vi "Html Report.vi"(0 "标题配置":cluster{"title":string, "font":T1}={"title"="测试报告", "font"={"font name"="", "font size"=24.0, "bold"=2, "italic"=2, "underline"=2, "strike through"=2, "font color"=16777222}} {"font"."font size" format="%0.2f"; "font"."strike through" items=["Unchanged", "Yes", "No"]; "font"."underline" items=["Unchanged", "Yes", "No"]; "font"."italic" items=["Unchanged", "Yes", "No"]; "font"."bold" items=["Unchanged", "Yes", "No"]}, 1 "测试信息":cluster{"font":T1, "字符串":string}={"font"={"font name"="", "font size"=12.0, "bold"=2, "italic"=2, "underline"=2, "strike through"=2, "font color"=16777222}, "字符串"=""} {"font"."font size" format="%0.2f"; "font"."strike through" items=["Strk Unchanged", "Strk Yes", "Strk No"]; "font"."underline" items=["Und Unchanged", "Und Yes", "Und No"]; "font"."italic" items=["Ital Unchanged", "Ital Yes", "Ital No"]; "font"."bold" items=["Bold Unchanged", "Bold Yes", "Bold No"]}, 2 "文本":cluster{"font":T1, "字符串":string}={"font"={"font name"="", "font size"=12.0, "bold"=2, "italic"=2, "underline"=2, "strike through"=2, "font color"=16777222}, "字符串"=""} {"font"."font size" format="%0.2f"; "font"."strike through" items=["Strk Unchanged", "Strk Yes", "Strk No"]; "font"."underline" items=["Und Unchanged", "Und Yes", "Und No"]; "font"."italic" items=["Ital Unchanged", "Ital Yes", "Ital No"]; "font"."bold" items=["Bold Unchanged", "Bold Yes", "Bold No"]}, 3 "表格":T2={"auto format"=11, "font"={"font name"="", "font size"=0.0, "bold"=0, "italic"=0, "underline"=0, "strike through"=0, "font color"=0}, "表格 2"=[["1", "1.5", "5.6", "5.6", "7.9", "4.6"], ["2", "2.5", "7.6", "6.5", "7.2", "7.5"], ["3", "6.8", "9.1", "4.2", "6.2", "6.1"], ["4", "6.7", "7.1", "7.2", "1.0", "8.3"], ["5", "6.4", "4.3", "9.2", "5.8", "4.2"], ["6", "8.6", "8.2", "4.3", "8.6", "4.5"]]} {"auto format" items=["xlRangeAutoFormat3DEffects1"=13, "xlRangeAutoFormat3DEffects2"=14, "xlRangeAutoFormatAccounting1"=4, "xlRangeAutoFormatAccounting2"=5, "xlRangeAutoFormatAccounting3"=6, "xlRangeAutoFormatAccounting4"=17, "xlRangeAutoFormatClassic1"=1, "xlRangeAutoFormatClassic2"=2, "xlRangeAutoFormatClassic3"=3, "xlRangeAutoFormatColor1"=7, "xlRangeAutoFormatColor2"=8, "xlRangeAutoFormatColor3"=9, "xlRangeAutoFormatList1"=10, "xlRangeAutoFormatList2"=11, "xlRangeAutoFormatList3"=12, "xlRangeAutoFormatLocalFormat1"=15, "xlRangeAutoFormatLocalFormat2"=16, "xlRangeAutoFormatLocalFormat3"=19, "xlRangeAutoFormatLocalFormat4"=20, "xlRangeAutoFormatReport1"=21, "xlRangeAutoFormatReport2"=22, "xlRangeAutoFormatReport3"=23, "xlRangeAutoFormatReport4"=24, "xlRangeAutoFormatReport5"=25, "xlRangeAutoFormatReport6"=26, "xlRangeAutoFormatReport7"=27, "xlRangeAutoFormatReport8"=28, "xlRangeAutoFormatReport9"=29, "xlRangeAutoFormatReport10"=30, "xlRangeAutoFormatClassicPivotTable"=31, "xlRangeAutoFormatTable1"=32, "xlRangeAutoFormatTable2"=33, "xlRangeAutoFormatTable3"=34, "xlRangeAutoFormatTable4"=35, "xlRangeAutoFormatTable5"=36, "xlRangeAutoFormatTable6"=37, "xlRangeAutoFormatTable7"=38, "xlRangeAutoFormatTable8"=39, "xlRangeAutoFormatTable9"=40, "xlRangeAutoFormatTable10"=41, "xlRangeAutoFormatPTNone"=42, "xlRangeAutoFormatNone"=-4142, "xlRangeAutoFormatSimple"=-4154]; "font"."font size" format="%0.2f"; "font"."strike through" items=["Strk Unchanged", "Strk Yes", "Strk No"]; "font"."underline" items=["Und Unchanged", "Und Yes", "Und No"]; "font"."italic" items=["Ital Unchanged", "Ital Yes", "Ital No"]; "font"."bold" items=["Bold Unchanged", "Bold Yes", "Bold No"]}, 4 "图表配置":T4={"chart type"=4, "graph title (\"\")"="测试图表"} {"chart type" items=["xlColumnClustered"=51, "xlColumnStacked"=52, "xlColumnStacked100"=53, "xl3DColumnClustered"=54, "xl3DColumnStacked"=55, "xl3DColumnStacked100"=56, "xlBarClustered"=57, "xlBarStacked"=58, "xlBarStacked100"=59, "xl3DBarClustered"=60, "xl3DBarStacked"=61, "xl3DBarStacked100"=62, "xlLineStacked"=63, "xlLineStacked100"=64, "xlLineMarkers"=65, "xlLineMarkersStacked"=66, "xlLineMarkersStacked100"=67, "xlPieOfPie"=68, "xlPieExploded"=69, "xl3DPieExploded"=70, "xlBarOfPie"=71, "xlXYScatterSmooth"=72, "xlXYScatterSmoothNoMarkers"=73, "xlXYScatterLines"=74, "xlXYScatterLinesNoMarkers"=75, "xlAreaStacked"=76, "xlAreaStacked100"=77, "xl3DAreaStacked"=78, "xl3DAreaStacked100"=79, "xlDoughnutExploded"=80, "xlRadarMarkers"=81, "xlRadarFilled"=82, "xlSurface"=83, "xlSurfaceWireframe"=84, "xlSurfaceTopView"=85, "xlSurfaceTopViewWireframe"=86, "xlBubble"=15, "xlBubble3DEffect"=87, "xlStockHLC"=88, "xlStockOHLC"=89, "xlStockVHLC"=90, "xlStockVOHLC"=91, "xlCylinderColClustered"=92, "xlCylinderColStacked"=93, "xlCylinderColStacked100"=94, "xlCylinderBarClustered"=95, "xlCylinderBarStacked"=96, "xlCylinderBarStacked100"=97, "xlCylinderCol"=98, "xlConeColClustered"=99, "xlConeColStacked"=100, "xlConeColStacked100"=101, "xlConeBarClustered"=102, "xlConeBarStacked"=103, "xlConeBarStacked100"=104, "xlConeCol"=105, "xlPyramidColClustered"=106, "xlPyramidColStacked"=107, "xlPyramidColStacked100"=108, "xlPyramidBarClustered"=109, "xlPyramidBarStacked"=110, "xlPyramidBarStacked100"=111, "xlPyramidCol"=112, "xl3DColumn"=-4100, "xlLine"=4, "xl3DLine"=-4101, "xl3DPie"=-4102, "xlPie"=5, "xlXYScatter"=-4169, "xl3DArea"=-4098, "xlArea"=1, "xlDoughnut"=-4120, "xlRadar"=-4151]}, 6 "报告类型":u16(ring)=2, 7 "簇":T3={"Save Report 2"=FALSE, "路径"=path "/Report.html", "Print Report 2"=FALSE, "份数"=1} {"份数" min=1 max=10 step=1}) -> ()   [LabVIEW 2014]
uses:
  <vilib>/addons/_office/_wordsub.llb/font.ctl
  <vilib>/Utility/NIReport.llb/Append Report Text (str wrap).vi
  <vilib>/printing/OpenHTMLReport.llb/Open HTML Report in Browser (Refnum).vi
  <vilib>/Utility/NIReport.llb/NI_report.lvclass
  <vilib>/Utility/NIReport.llb/NI_ReportGenerationCore.lvlib
panel:
  out "表格 2":string[][](table)=[["1", "1.5", "5.6", "5.6", "7.9", "4.6"], ["2", "2.5", "7.6", "6.5", "7.2", "7.5"], ["3", "6.8", "9.1", "4.2", "6.2", "6.1"], ["4", "6.7", "7.1", "7.2", "1.0", "8.3"], ["5", "6.4", "4.3", "9.2", "5.8", "4.2"], ["6", "8.6", "8.2", "4.3", "8.6", "4.5"]]
  out "波形图":i32[][](graph)
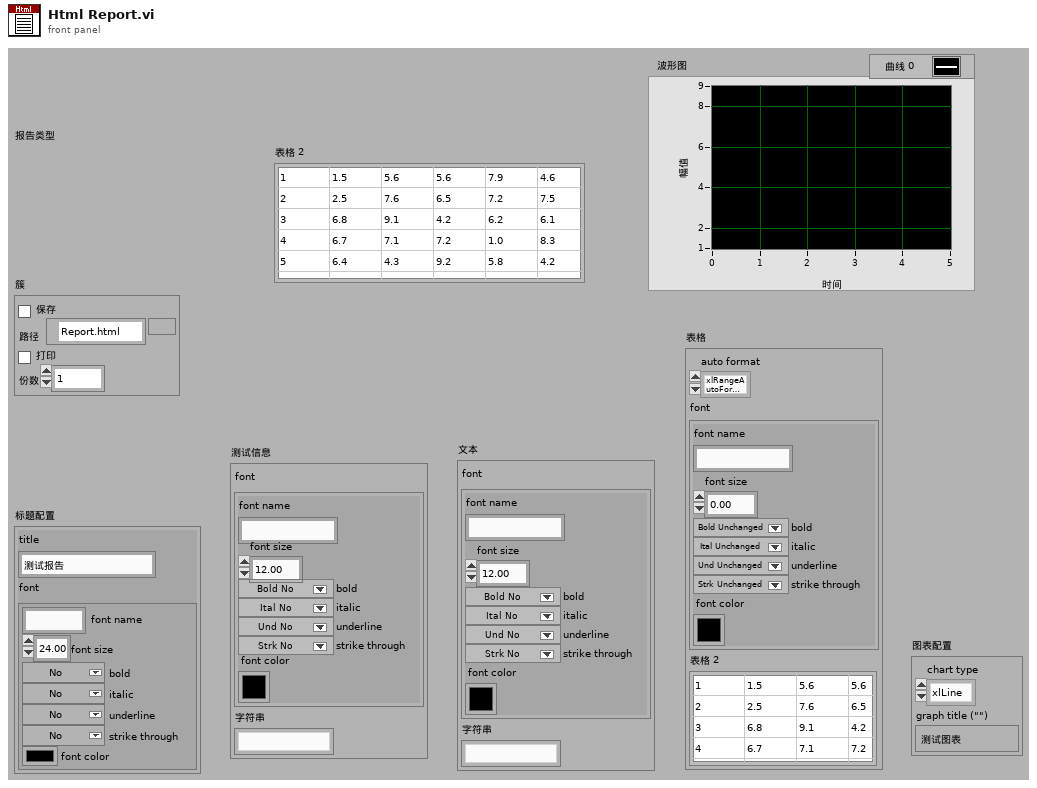
[diagram p1: front panel]
types:
  T1 = typedef "font.ctl" = cluster{"font name":string, "font size":dbl, "bold":u16, "italic":u16, "underline":u16, "strike through":u16, "font color":u32}
  T2 = cluster{"auto format":i32, "font":T1, "表格 2":string[][]}
  T3 = cluster{"Save Report 2":bool, "路径":path, "Print Report 2":bool, "份数":i32}
  T4 = cluster{"chart type":i32, "graph title (\"\")":string}
  T5 = cluster{"Charset (-1)":i16, "Weight (-1)":i16, "Name":string, "Size":string}
  T6 = cluster{"Italic":enum16{"Italic Unchanged", "Italic On", "Italic Off"}, "Strike Through":enum16{"Strike Through Unchanged", "Strike Through On", "Strike Through Off"}, "Underline":enum16{"Underline Unchanged", "Underline On", "Underline Off"}, "Bold":enum16{"Bold Unchanged", "Bold On", "Bold Off"}}
  T7 = typedef "Generate Report Object Reference.ctl" = refnum<class "NI_report.lvclass">
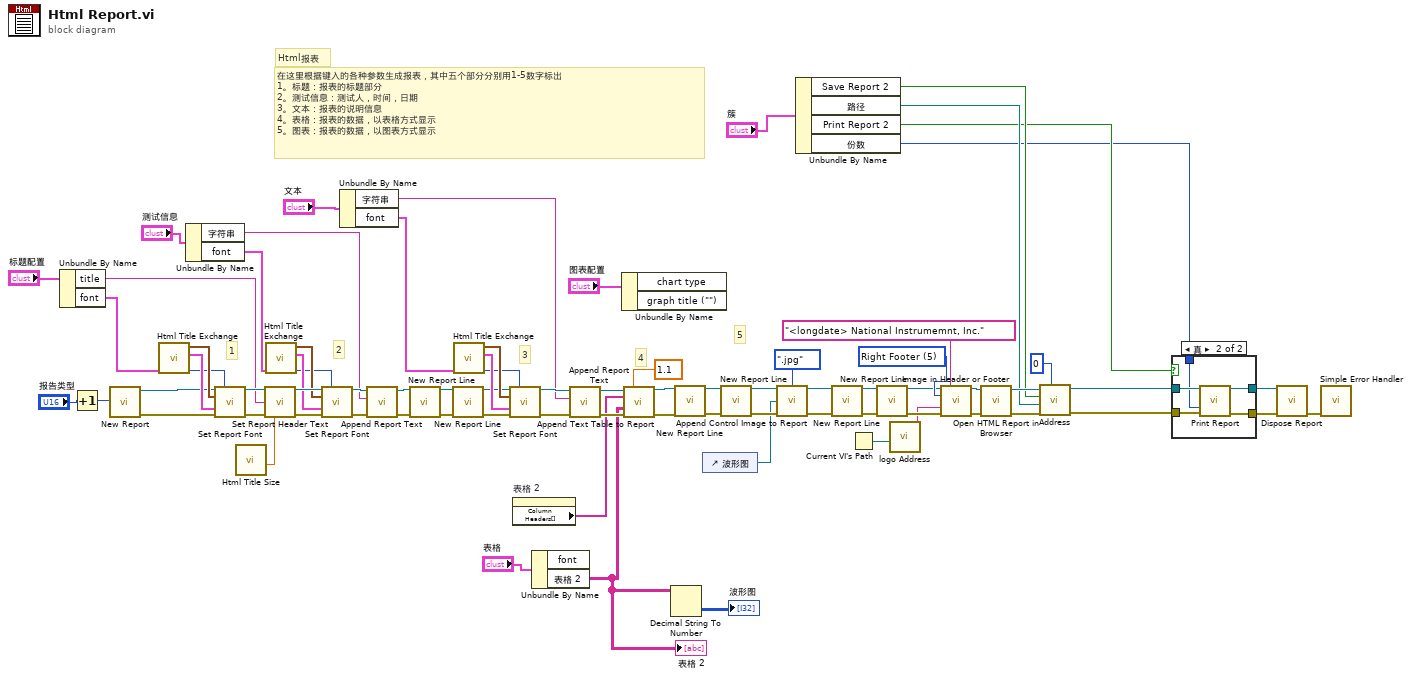
[diagram p0: block diagram]
diagram:
  w64 = u16 5 items=["Left Header", "Left Footer", "Center Header", "Center Footer", "Right Herader", "Right Footer"] ("select header or footer")
  # "3"
  # "2"
  # "5"
  # "4"
  # "1"
  # "Html报表"
  # "在这里根据键入的各种参数生成报表，其中五个部分分别用1-5数字标出\n1。标题：报表的标题部分\n2。测试信息：测试人，时间，日期\n3。文本：报表的说明信息\n4。表格：报表的数据，以表格方式显示\n5。图表：报表的数据，以图表方式显示"
  n1 = Unbundle By Name("标题配置") -> ("title"=w14:string, "font"=w15:T1)
  n2 = Increment(x="报告类型") -> (x+1=w74:u16)
  n3 = call <vilib>:"New Report.vi"("report type"=w74) -> ("report out"=w17:refnum<class "NI_report.lvclass">, "error out"=w16:errorcluster)  [unwired: 13 in]
  n4 = call "Html Title Exchange.vi"("font"=w15) -> ("text color (unchanged)"=w39:u32, "font settings"=w65:T5, "text options"=w66:T6)  [unwired: 8 in]
  n5 = Unbundle By Name("测试信息") -> ("字符串"=w12:string, "font"=w13:T1)
  n6 = call-dynamic "Set Report Font.vi"("report in"=w17, "text color (unchanged)"=w39, "text options"=w66, "font settings"=w65, "error in (no error)"=w16) -> ("report out"=w67:refnum<class "NI_report.lvclass">, "error out"=w68:errorcluster)  [unwired: 8 in, 1 out]
  n7 = call "Html Title Size.vi"() -> ("数值"=w42:dbl)  [unwired: 11 in]
  n8 = call-dynamic "Set Report Header Text.vi"("report in"=w67, "center header text"=w14, "error in (no error)"=w68, "HTML header size"=w42) -> ("report out"=w69:refnum<class "NI_report.lvclass">, "error out"=w70:errorcluster)  [unwired: 10 in]
  n9 = call "Html Title Exchange.vi"("font"=w13) -> ("text color (unchanged)"=w38:u32, "font settings"=w40:T5, "text options"=w41:T6)  [unwired: 8 in]
  n10 = call-dynamic "Set Report Font.vi"("report in"=w69, "text color (unchanged)"=w38, "text options"=w41, "font settings"=w40, "error in (no error)"=w70) -> ("report out"=w71:refnum<class "NI_report.lvclass">, "error out"=w28:errorcluster)  [unwired: 8 in, 1 out]
  n11 = Unbundle By Name("文本") -> ("字符串"=w11:string, "font"=w10:T1)
  n12 = call-poly <vilib>:"Append Report Text.vi"("report in"=w71, "text"=w12, "error in (no error)"=w28) -> ("report out"=w49:refnum<class "NI_report.lvclass">, "error out"=w50:errorcluster)  [unwired: 9 in, 2 out]
  n13 = call-dynamic "New Report Line.vi"("report in"=w49, "error in (no error)"=w50) -> ("report out"=w32:refnum<class "NI_report.lvclass">, "error out"=w29:errorcluster)  [unwired: 12 in]
  n14 = call-dynamic "New Report Line.vi"("report in"=w32, "error in (no error)"=w29) -> ("report out"=w31:refnum<class "NI_report.lvclass">, "error out"=w30:errorcluster)  [unwired: 12 in]
  n15 = call "Html Title Exchange.vi"("font"=w10) -> ("text color (unchanged)"=w33:u32, "font settings"=w34:T5, "text options"=w35:T6)  [unwired: 8 in]
  n16 = call-dynamic "Set Report Font.vi"("report in"=w31, "text color (unchanged)"=w33, "text options"=w35, "font settings"=w34, "error in (no error)"=w30) -> ("report out"=w51:refnum<class "NI_report.lvclass">, "error out"=w52:errorcluster)  [unwired: 8 in, 1 out]
  n17 = property on="表格 2" class="Tbl (严格)"() -> ("Column Headers[]"=w8:string[])  [unwired: 2 in, 2 out]
  n18 = Unbundle By Name("表格") -> ("表格 2"=w7:string[][])  [unwired: 1 out]
  "表格 2" <- w7
  n19 = call-poly <vilib>:"Append Report Text.vi"("report in"=w51, "text"=w11, "error in (no error)"=w52) -> ("report out"=w48:refnum<class "NI_report.lvclass">, "error out"=w47:errorcluster)  [unwired: 9 in, 2 out]
  n20 = Unbundle By Name("图表配置") -> ()  [unwired: 2 out]
  n21 = call-dynamic "Append Text Table to Report.vi"("report in"=w48, "column width (1)"=1.1, "column headers"=w8, "text data"=w7, "error in (no error)"=w47) -> ("report out"=w62:refnum<class "NI_report.lvclass">, "error out"=w61:errorcluster)  [unwired: 7 in, 2 out]
  n22 = Decimal String To Number(string=w7) -> (number=→"波形图":i32[][])  [unwired: 2 in, 1 out]
  n23 = call-dynamic "New Report Line.vi"("report in"=w62, "error in (no error)"=w61) -> ("report out"=w45:refnum<class "NI_report.lvclass">, "error out"=w46:errorcluster)  [unwired: 12 in]
  n24 = control-ref of="波形图"() -> (w5:refnum<vi>)
  n25 = call-dynamic "New Report Line.vi"("report in"=w45, "error in (no error)"=w46) -> ("report out"=w53:refnum<class "NI_report.lvclass">, "error out"=w54:errorcluster)  [unwired: 12 in]
  n26 = call-dynamic "Append Control Image to Report.vi"("report in"=w53, "image file type (.jpg)"=enum16{".jpg", ".png"}.".jpg" ("image file type(.png)"), "ctrl reference"=w5, "error in (no error)"=w54) -> ("report out"=w56:refnum<class "NI_report.lvclass">, "error out"=w57:errorcluster)  [unwired: 8 in, 2 out]
  n27 = Unbundle By Name("簇") -> ("Save Report 2"=w4:bool, "路径"=w3:path, "Print Report 2"=w2:bool, "份数"=w1:i32)
  n28 = call-dynamic "New Report Line.vi"("report in"=w56, "error in (no error)"=w57) -> ("report out"=w60:refnum<class "NI_report.lvclass">, "error out"=w59:errorcluster)  [unwired: 12 in]
  n29 = Current VI's Path() -> (path=w24:path)
  n30 = call-dynamic "New Report Line.vi"("report in"=w60, "error in (no error)"=w59) -> ("report out"=w44:refnum<class "NI_report.lvclass">, "error out"=w43:errorcluster)  [unwired: 12 in]
  n31 = call "logo Address.vi"("path"=w24) -> ("字符串"=w23:string)  [unwired: 10 in]
  n32 = call-dynamic "Image in Header or Footer.vi"("report in"=w44, "select header or footer"=w64, "image path"=w23, "error in (no error)"=w43, "text above image"="<longdate> National Instrumemnt, Inc." ("right footer text")) -> ("report out"=w36:refnum<class "NI_report.lvclass">, "error out"=w37:errorcluster)  [unwired: 9 in]
  n33 = call-poly <vilib>:"Open HTML Report in Browser.vi"("report in"=w36, "error in (no error)"=w37) -> ("report out"=w22:refnum<class "NI_report.lvclass">, "error out"=w21:errorcluster)  [unwired: 11 in, 1 out]
  n34 = call "Address.vi"("报告类型"=u16 0 ("报告类型 2"), "错误簇输入"=w21, "路径"=w3, "保存？"=w4, "报告输入"=w22) -> ("错误簇输出"=w20:errorcluster, "报告输出"=w19:T7)  [unwired: 5 in]
  n35 = case shown="真" w2 {
    tunnel: [w80 w84] -> w27
    tunnel: [w79 w85] -> w26
    tunnel: w20 -> [w79 w83]
    tunnel: w19 -> [w80 w82]
    tunnel: w1 -> [_ w81]
    frame False {
    }
    frame True {
      n36 = call-dynamic "Print Report.vi"("report in"=w82, "number of copies (1)"=w81, "error in (no error)"=w83) -> ("report out"=w84:T7, "error out"=w85:errorcluster)  [unwired: 11 in]
    }
  }
  n37 = call-dynamic "Dispose Report.vi"("report in"=w27, "error in (no error)"=w26) -> ("error out"=w25:errorcluster)  [unwired: 13 in]
  n38 = call <vilib>:"Simple Error Handler.vi"("error in (no error)"=w25) -> ()  [unwired: 4 in, 5 out]
